vi "PXI-Start AOAI.vi"(0 "AO Tasks":T1[](array[typedef]), 1 "DI Tasks":T1[](array[typedef]), 2 "DO Tasks":T1[](array[typedef]), 5 "AI Tasks":T1[](array[typedef]), 7 "Counter Task":T1, 9 "Sync Task":T1, 11 "error in (no error)":errorcluster) -> (4 "AO Tasks out":T1[](array[typedef]), 15 "error out":errorcluster)   [LabVIEW 2020]
uses:
  Type Defs/Task Struct.ctl
  PXI Globals.vi
  <resource>/objmgr/daqmx.rc
panel:
  out "Sync Task out":T1
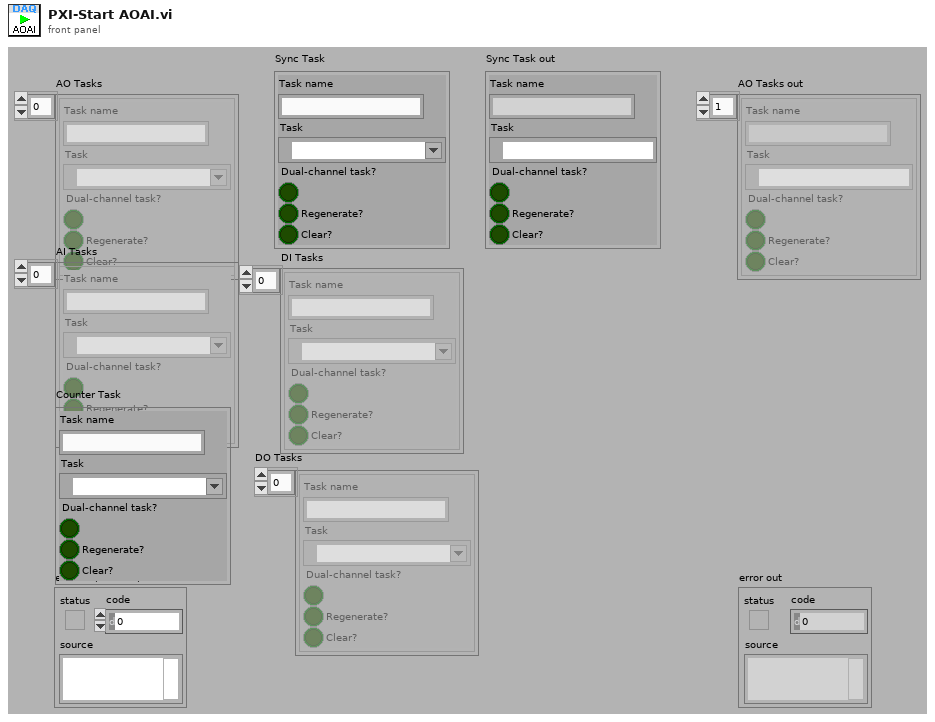
[diagram p1: front panel]
types:
  T1 = typedef "Task Struct.ctl" = cluster{"Task name":string, "Task":refnum<k21>, "Dual-channel task?":bool, "Regenerate?":bool, "Clear?":bool}
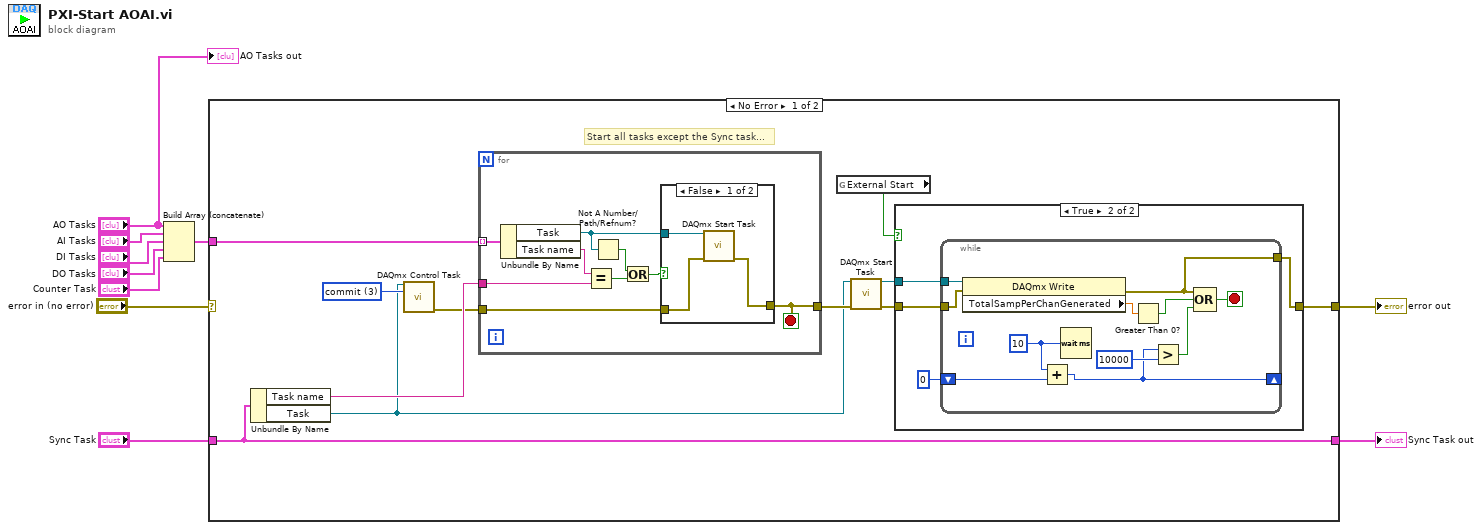
[diagram p0: block diagram]
diagram:
  n1 = Build Array (concatenate)("AO Tasks", "AI Tasks", "DI Tasks", "DO Tasks", "Counter Task") -> (w3:T1[])
  n2 = case shown="No Error" "error in (no error)" {
    selector: "error in (no error)" -> [_ w50]
    tunnel: [w15 w50] -> w10
    tunnel: "Sync Task" -> [w20 w51]
    tunnel: [w20 w51] -> w8
    tunnel: w3 -> [w19 _]
    frame No Error {
      w13 = 3 items=["verify"=2, "reserve"=4, "commit"=3, "unreserve"=5, "abort"=6] ("action")
      # "Start all tasks except the Sync task..."
      n3 = Unbundle By Name(w20) -> ("Task name"=w21:string, "Task"=w12:refnum<k21>)
      n4 = call <vilib>:"DAQmx Control Task.vi"("task/channels in"=w12, "action"=w13) -> ("error out"=w11:errorcluster)  [unwired: 12 in, 1 out]
      n5 = for {
        tunnel: w19 -> [w30] mode=indexing
        tunnel: w21 -> [w27]
        tunnel: [w26] -> w18
        tunnel: w11 -> [w22]
        stop <- w26 stop-if-true
        n6 = Unbundle By Name(w30) -> ("Task"=w25:refnum<k21>, "Task name"=w28:string)
        n7 = Equal?(x=w28, y=w27) -> (x = y?=w29:bool)
        n8 = Not A Number/Path/Refnum?(number/path/refnum=w25) -> (NaN/Path/Refnum?=w23:bool)
        n9 = Or(x=w23, y=w29) -> (x .or. y?=w24:bool)
        n10 = case shown="False" w24 {
          tunnel: w25 -> [w33 _]
          tunnel: [w32 _] -> w26
          tunnel: w22 -> [w31 _]
          frame False {
            n11 = call <vilib>:"DAQmx Start Task.vi"("task/channels in"=w33, "error in"=w31) -> ("error out"=w32:errorcluster)  [unwired: 12 in, 1 out]
          }
          frame True {
            # "Don't start\nthe Sync task"
          }
        }
      }
      n12 = global read "PXI Globals.vi" "External Start"() -> (w14:bool)
      n13 = call <vilib>:"DAQmx Start Task.vi"("task/channels in"=w12, "error in"=w18) -> ("task out"=w16:refnum<k21>, "error out"=w17:errorcluster)  [unwired: 12 in]
      n14 = case shown="True" w14 {
        tunnel: w17 -> [w34 w38]
        tunnel: w16 -> [_ w37]
        tunnel: [w34 w35] -> w15
        frame False {
        }
        frame True {
          n15 = while {
            tunnel: w38 -> [w48]
            tunnel: w37 -> [w49]
            shift-right: [w40] -> _
            shift-left: 0 -> [w44]
            tunnel: [w39] -> w35
            stop <- w45 stop-if-true
            w41 = u32 10 ("milliseconds to wait")
            n16 = property class="DAQmx Write"(reference=w49, error in=w48) -> (error out=w39:errorcluster, "TotalSampPerChanGenerated"=w47:dbl)  [unwired: 1 out]
            n17 = Add(x=w41, y=w44) -> (x+y=w40:u32)
            n18 = Wait (ms)(milliseconds to wait=w41) -> ()  [unwired: 1 out]
            n19 = Greater Than 0?(x=w47) -> (x > 0?=w46:bool)
            n20 = Greater?(x=w40, y=10000) -> (0:w42:bool)
            n21 = Compound Arithmetic op=OR(w39, w46, w42) -> (w45:bool)
          }
        }
      }
    }
    frame Error {
    }
  }
  "error out" <- w10
  "Sync Task out" <- w8
  "AO Tasks out" <- "AO Tasks"
